vi "Lab Panel V5.25.vi"() -> ()   [LabVIEW 2017] (continued)
                        n582 = Unbundle(w867) -> ("AMPS"=w870:dbl)  [unwired: 4 out]
                        n583 = call "Check For Amps on v1.vi"("ID"="LAB01-2", "amps"=w870) -> ("amps"=w868:bool)  [unwired: 9 in]
                      }
                      frame #1 {
                        n584 = case shown="True" w872 {
                          tunnel: w882 -> [_ w895]
                          tunnel: w881 -> [_ w894]
                          tunnel: w880 -> [_ w893]
                          tunnel: w879 -> [_ w892]
                          tunnel: w878 -> [_ w891]
                          tunnel: [errorcluster {"status"=FALSE, "code"=0, "source"=""} ("error out") w890] -> w877
                          tunnel: w876 -> [_ w889]
                          tunnel: w875 -> [_ w888]
                          tunnel: w874 -> [_ w887]
                          tunnel: w873 -> [_ w886]
                          tunnel: w871 -> [_ w885]
                          frame False {
                            w883 = FALSE
                            n585 = local write "RUN LAB01-2"(w883) -> ()
                            n586 = local write "run lab01-2"(w883) -> ()
                          }
                          frame True {
                            n587 = stacked-sequence {
                              seq-local: [w896 _ _ _ _] -> [_ w920 _ _ _]
                              tunnel: w895 -> [w901 _ _ _ _]
                              tunnel: w894 -> [w898 _ _ _ _]
                              tunnel: w893 -> [w911 _ _ _ _]
                              tunnel: w892 -> [w904 _ _ _ _]
                              tunnel: w891 -> [w899 _ _ _ _]
                              tunnel: [_ w915 _ _ _] -> w890
                              tunnel: w889 -> [_ _ _ w942 _]
                              tunnel: w888 -> [_ _ _ w941 _]
                              tunnel: w887 -> [_ _ _ w940 _]
                              tunnel: w886 -> [_ _ _ _ _]
                              tunnel: w885 -> [_ _ _ _ w955]
                              frame #0 {
                                w897 = "\\"
                                n588 = local read "SET LAB01-2"() -> (w906:T5)
                                n589 = case shown="\"CYCLE TEST\"" w911 {
                                tunnel: ["L01-2-CHART TEST-" "L01-2-CYCLE TEST-" "L01-2-T-RISE TEST-"] -> w907
                                frame "CHART TEST", Default {
                                }
                                frame "CYCLE TEST" {
                                }
                                frame "T-RISE TEST" {
                                }
                                }
                                n590 = Unbundle(w906) -> ("DESCRIPTION"=w905:string)  [unwired: 4 out]
                                n591 = Concatenate Strings(w901, "\\", w899, w897, w898, w897) -> (w908:string)
                                n592 = String To Path(string=w908) -> (path=w910:path)
                                n593 = Concatenate Strings(w908, w907, w905, "-", w904, ".tdms") -> (w896:string)
                                n594 = Create Folder(path (use dialog)=w910) -> (error out=w909:errorcluster)  [unwired: 2 in, 2 out]
                                n595 = call <vilib>:"Clear Errors.vi"("error in (no error)"=w909) -> ()  [unwired: 5 in, 2 out]
                                n596 = global write "Global 1.vi" "LAB01-2 FILE"(w896) -> ()
                              }
                              frame #1 {
                                (unwired) FALSE
                                n597 = String To Path(string=w920) -> (path=w916:path)
                                n598 = TDMS Open(6:FALSE, 10:T21."create or replace" ("operation (0:open)"), 11:w916) -> (0:w915:errorcluster, 3:→"TDMS LAB01-2":refnum<k34>)  [unwired: 4 in]
                              }
                              frame #2 {
                                n599 = local read "SET LAB01-2"() -> (w926:T5)
                                n600 = local read "TDMS LAB01-2"() -> (w937:refnum<k34>)
                                n601 = Build Array("Testers Name", "Description", "Set Test Cycles", "T-Rise minutes", "T-Rise Deg C") -> (w927:string[])
                                n602 = Unbundle(w926) -> ("NAME"=w925:string, "DESCRIPTION"=w924:string, "CYCLES"=w923:dbl, "T-RISE mins"=w922:dbl, "T-RISE deg C"=w921:dbl)
                                n603 = Number To Decimal String(number=w923) -> (decimal integer string=w936:string)  [unwired: 1 in]
                                n604 = Number To Decimal String(number=w922) -> (decimal integer string=w935:string)  [unwired: 1 in]
                                n605 = Number To Decimal String(number=w921) -> (decimal integer string=w934:string)  [unwired: 1 in]
                                n606 = Build Array(w925, w924, w936, w935, w934) -> (w933:string[])
                                n607 = TDMS Set Properties(5:w933, 7:w927, 11:w937) -> ()  [unwired: 3 in, 4 out]
                              }
                              frame #3 {
                                n608 = local read "DISP LAB01-2"() -> (w939:T4)
                                n609 = Concatenate Strings("LAB01-2  ", w942) -> (w943:string)
                                n610 = Two Button Dialog(message=w943, 1:w940, 2:w941) -> (T button?=w945:bool)
                                n611 = case shown="True" w945 {
                                tunnel: w939 -> [w952 w953]
                                tunnel: [w952 w953] -> w949
                                tunnel: [w951 w954] -> w948
                                tunnel: [w950 w954] -> w947
                                frame False {
                                n612 = Unbundle(w952) -> ("CYCLE"=w951:dbl, "MINS"=w950:dbl)  [unwired: 1 out]
                                }
                                frame True {
                                w954 = 0.0
                                }
                                }
                                n613 = Bundle(cluster=w949, "CYCLE"=w948, "MINS"=w947, "STATUS"="RUN") -> (w938:T4)
                                n614 = local write "DISP LAB01-2"(w938) -> ()
                              }
                              frame #4 {
                                n615 = local read "TEMP START LAB01-2"() -> (w957:cluster{"TL":dbl, "TN":dbl})
                                n616 = Bundle(cluster=w957, "TL"=w955, "TN"=w955) -> (w956:cluster{"TL":dbl, "TN":dbl})
                                n617 = local write "TEMP START LAB01-2"(w956) -> ()
                              }
                            }
                          }
                        }
                      }
                    }
                  }
                }
              }
              event "RUN LAB02-1": Value Change {
                n618 = event-data() -> ("NewVal"=w963:bool)  [unwired: 1 in, 5 out]
                n619 = local read "SIG LAB02-1"() -> (w959:T2)
                n620 = case shown="True" w963 {
                  tunnel: w969 -> [_ w1007]
                  tunnel: w968 -> [_ w1006]
                  tunnel: w966 -> [w971 w1005]
                  tunnel: w967 -> [_ w1004]
                  tunnel: w965 -> [_ w1003]
                  tunnel: [w970 w1002] -> w964
                  tunnel: w962 -> [_ w1001]
                  tunnel: w961 -> [_ w1000]
                  tunnel: w960 -> [_ w999]
                  tunnel: w959 -> [_ w998]
                  tunnel: w958 -> [_ w997]
                  frame False {
                    # "stop test"
                    n621 = stacked-sequence {
                      tunnel: w971 -> [w980 _]
                      tunnel: [w972 _] -> w970
                      frame #0 {
                        n622 = local read "DISP LAB02-1"() -> (w979:T4)
                        n623 = Unbundle(w979) -> ("CYCLE"=w977:dbl, "MINS"=w978:dbl)  [unwired: 1 out]
                        n624 = case shown="\"CYCLE TEST\"" w980 {
                          tunnel: w978 -> [_ _ w987]
                          tunnel: w977 -> [w985 w986 _]
                          tunnel: [w985 w986 w987] -> w976
                          frame "CHART TEST", Default {
                          }
                          frame "CYCLE TEST" {
                          }
                          frame "T-RISE TEST" {
                          }
                        }
                        n625 = local read "TDMS LAB02-1"() -> (w984:refnum<k34>)
                        n626 = Build Array("STOPPED") -> (w981:string[])
                        n627 = Build Array(w976) -> (w975:dbl[])
                        n628 = TDMS Write(0:w984, 5:"TEST RESULT", 7:w981, 9:w975) -> (4:w973:refnum<k34>, 15:w974:errorcluster)  [unwired: 2 in, 2 out]
                        n629 = TDMS Close(8:w974, 11:w973) -> (0:w972:errorcluster)  [unwired: 1 out]
                      }
                      frame #1 {
                        n630 = local read "DISP LAB02-1"() -> (w991:T4)
                        n631 = stacked-sequence {
                          tunnel: "LAB02-1" -> [w993 w995]
                          frame #0 {
                            n632 = call "sub vi - defrag tdms v1.vi"("panel id"=w993) -> ("error out"=w992:errorcluster)  [unwired: 10 in]
                            n633 = local write "data file error"(w992) -> ()
                          }
                          frame #1 {
                            n634 = local write "RESULT LAB02-1"(FALSE) -> ()
                            n635 = call "Save data file (stop) v3.vi"("panel id"=w995) -> ("network file save error"=w994:errorcluster)  [unwired: 9 in, 1 out]
                            n636 = local write "data file error"(w994) -> ()
                          }
                        }
                        n637 = Bundle(cluster=w991, "STATUS"="STOP") -> (w989:T4)  [unwired: 2 in]
                        n638 = local write "DISP LAB02-1"(w989) -> ()
                      }
                    }
                  }
                  frame True {
                    n639 = stacked-sequence {
                      seq-local: [w1009 _] -> [_ w1013]
                      tunnel: w1007 -> [_ w1023]
                      tunnel: w1006 -> [_ w1022]
                      tunnel: w1005 -> [_ w1021]
                      tunnel: w1004 -> [_ w1020]
                      tunnel: w1003 -> [_ w1019]
                      tunnel: [_ w1018] -> w1002
                      tunnel: w1001 -> [_ w1017]
                      tunnel: w1000 -> [_ w1016]
                      tunnel: w999 -> [_ w1015]
                      tunnel: w998 -> [w1008 w1014]
                      tunnel: w997 -> [_ w1012]
                      frame #0 {
                        n640 = Unbundle(w1008) -> ("AMPS"=w1011:dbl)  [unwired: 4 out]
                        n641 = call "Check For Amps on v1.vi"("ID"="LAB02-1", "amps"=w1011) -> ("amps"=w1009:bool)  [unwired: 9 in]
                      }
                      frame #1 {
                        n642 = case shown="True" w1013 {
                          tunnel: w1023 -> [_ w1036]
                          tunnel: w1022 -> [_ w1035]
                          tunnel: w1021 -> [_ w1034]
                          tunnel: w1020 -> [_ w1033]
                          tunnel: w1019 -> [_ w1032]
                          tunnel: [errorcluster {"status"=FALSE, "code"=0, "source"=""} ("error out") w1031] -> w1018
                          tunnel: w1017 -> [_ w1030]
                          tunnel: w1016 -> [_ w1029]
                          tunnel: w1015 -> [_ w1028]
                          tunnel: w1014 -> [_ w1027]
                          tunnel: w1012 -> [_ w1026]
                          frame False {
                            w1025 = FALSE
                            n643 = local write "RUN LAB02-1"(w1025) -> ()
                            n644 = local write "run lab02-1"(w1025) -> ()
                          }
                          frame True {
                            n645 = stacked-sequence {
                              seq-local: [w1037 _ _ _ _] -> [_ w1061 _ _ _]
                              tunnel: w1036 -> [w1042 _ _ _ _]
                              tunnel: w1035 -> [w1039 _ _ _ _]
                              tunnel: w1034 -> [w1052 _ _ _ _]
                              tunnel: w1033 -> [w1045 _ _ _ _]
                              tunnel: w1032 -> [w1040 _ _ _ _]
                              tunnel: [_ w1056 _ _ _] -> w1031
                              tunnel: w1030 -> [_ _ _ w1082 _]
                              tunnel: w1029 -> [_ _ _ w1081 _]
                              tunnel: w1028 -> [_ _ _ w1080 _]
                              tunnel: w1027 -> [_ _ _ _ _]
                              tunnel: w1026 -> [_ _ _ _ w1096]
                              frame #0 {
                                w1038 = "\\"
                                n646 = local read "SET LAB02-1"() -> (w1047:T5)
                                n647 = case shown="\"CYCLE TEST\"" w1052 {
                                tunnel: ["L02-1-CHART TEST-" "L02-1-CYCLE TEST-" "L02-1-T-RISE TEST-"] -> w1048
                                frame "CHART TEST", Default {
                                }
                                frame "CYCLE TEST" {
                                }
                                frame "T-RISE TEST" {
                                }
                                }
                                n648 = Unbundle(w1047) -> ("DESCRIPTION"=w1046:string)  [unwired: 4 out]
                                n649 = Concatenate Strings(w1042, "\\", w1040, w1038, w1039, w1038) -> (w1049:string)
                                n650 = String To Path(string=w1049) -> (path=w1051:path)
                                n651 = Concatenate Strings(w1049, w1048, w1046, "-", w1045, ".tdms") -> (w1037:string)
                                n652 = Create Folder(path (use dialog)=w1051) -> (error out=w1050:errorcluster)  [unwired: 2 in, 2 out]
                                n653 = global write "Global 1.vi" "LAB02-1 FILE"(w1037) -> ()
                                n654 = call <vilib>:"Clear Errors.vi"("error in (no error)"=w1050) -> ()  [unwired: 5 in, 2 out]
                              }
                              frame #1 {
                                (unwired) FALSE
                                n655 = String To Path(string=w1061) -> (path=w1057:path)
                                n656 = TDMS Open(6:FALSE, 10:T21."create or replace" ("operation (0:open)"), 11:w1057) -> (0:w1056:errorcluster, 3:→"TDMS LAB02-1":refnum<k34>)  [unwired: 4 in]
                              }
                              frame #2 {
                                n657 = local read "SET LAB02-1"() -> (w1067:T5)
                                n658 = local read "TDMS LAB02-1"() -> (w1078:refnum<k34>)
                                n659 = Build Array("Testers Name", "Description", "Set Test Cycles", "T-Rise minutes", "T-Rise Deg C") -> (w1068:string[])
                                n660 = Unbundle(w1067) -> ("NAME"=w1066:string, "DESCRIPTION"=w1065:string, "CYCLES"=w1064:dbl, "T-RISE mins"=w1063:dbl, "T-RISE deg C"=w1062:dbl)
                                n661 = Number To Decimal String(number=w1064) -> (decimal integer string=w1077:string)  [unwired: 1 in]
                                n662 = Number To Decimal String(number=w1063) -> (decimal integer string=w1076:string)  [unwired: 1 in]
                                n663 = Number To Decimal String(number=w1062) -> (decimal integer string=w1075:string)  [unwired: 1 in]
                                n664 = Build Array(w1066, w1065, w1077, w1076, w1075) -> (w1074:string[])
                                n665 = TDMS Set Properties(5:w1074, 7:w1068, 11:w1078) -> ()  [unwired: 3 in, 4 out]
                              }
                              frame #3 {
                                n666 = local read "DISP LAB02-1"() -> (w1083:T4)
                                n667 = Concatenate Strings("LAB02-1  ", w1082) -> (w1084:string)
                                n668 = Two Button Dialog(message=w1084, 1:w1080, 2:w1081) -> (T button?=w1086:bool)
                                n669 = case shown="True" w1086 {
                                tunnel: w1083 -> [w1093 w1094]
                                tunnel: [w1093 w1094] -> w1090
                                tunnel: [w1092 w1095] -> w1089
                                tunnel: [w1091 w1095] -> w1088
                                frame False {
                                n670 = Unbundle(w1093) -> ("CYCLE"=w1092:dbl, "MINS"=w1091:dbl)  [unwired: 1 out]
                                }
                                frame True {
                                w1095 = 0.0
                                }
                                }
                                n671 = Bundle(cluster=w1090, "CYCLE"=w1089, "MINS"=w1088, "STATUS"="RUN") -> (w1079:T4)
                                n672 = local write "DISP LAB02-1"(w1079) -> ()
                              }
                              frame #4 {
                                n673 = local read "TEMP START LAB02-1"() -> (w1098:cluster{"TL":dbl, "TN":dbl})
                                n674 = Bundle(cluster=w1098, "TL"=w1096, "TN"=w1096) -> (w1097:cluster{"TL":dbl, "TN":dbl})
                                n675 = local write "TEMP START LAB02-1"(w1097) -> ()
                              }
                            }
                          }
                        }
                      }
                    }
                  }
                }
                n676 = local write "run lab02-1"(w963) -> ()
              }
              event "RUN LAB02-2": Value Change {
                n677 = event-data() -> ("NewVal"=w1103:bool)  [unwired: 1 in, 5 out]
                n678 = local write "run lab02-2"(w1103) -> ()
                n679 = case shown="True" w1103 {
                  tunnel: w1109 -> [_ w1147]
                  tunnel: w1108 -> [_ w1146]
                  tunnel: w1106 -> [w1111 w1145]
                  tunnel: w1107 -> [_ w1144]
                  tunnel: w1105 -> [_ w1143]
                  tunnel: [w1110 w1142] -> w1104
                  tunnel: w1102 -> [_ w1141]
                  tunnel: w1101 -> [_ w1140]
                  tunnel: w1100 -> [_ w1139]
                  tunnel: w1099 -> [_ w1137]
                  frame False {
                    # "stop test"
                    n680 = stacked-sequence {
                      tunnel: w1111 -> [w1120 _]
                      tunnel: [w1112 _] -> w1110
                      frame #0 {
                        n681 = local read "DISP LAB02-2"() -> (w1119:T4)
                        n682 = Unbundle(w1119) -> ("CYCLE"=w1117:dbl, "MINS"=w1118:dbl)  [unwired: 1 out]
                        n683 = case shown="\"CYCLE TEST\"" w1120 {
                          tunnel: w1118 -> [_ _ w1127]
                          tunnel: w1117 -> [w1125 w1126 _]
                          tunnel: [w1125 w1126 w1127] -> w1116
                          frame "CHART TEST", Default {
                          }
                          frame "CYCLE TEST" {
                          }
                          frame "T-RISE TEST" {
                          }
                        }
                        n684 = local read "TDMS LAB02-2"() -> (w1124:refnum<k34>)
                        n685 = Build Array("STOPPED") -> (w1121:string[])
                        n686 = Build Array(w1116) -> (w1115:dbl[])
                        n687 = TDMS Write(0:w1124, 5:"TEST RESULT", 7:w1121, 9:w1115) -> (4:w1113:refnum<k34>, 15:w1114:errorcluster)  [unwired: 2 in, 2 out]
                        n688 = TDMS Close(8:w1114, 11:w1113) -> (0:w1112:errorcluster)  [unwired: 1 out]
                      }
                      frame #1 {
                        n689 = local read "DISP LAB02-2"() -> (w1131:T4)
                        n690 = stacked-sequence {
                          tunnel: "LAB02-2" -> [w1133 w1135]
                          frame #0 {
                            n691 = call "sub vi - defrag tdms v1.vi"("panel id"=w1133) -> ("error out"=w1132:errorcluster)  [unwired: 10 in]
                            n692 = local write "data file error"(w1132) -> ()
                          }
                          frame #1 {
                            n693 = call "Save data file (stop) v3.vi"("panel id"=w1135) -> ("network file save error"=w1134:errorcluster)  [unwired: 9 in, 1 out]
                            n694 = local write "RESULT LAB02-2"(FALSE) -> ()
                            n695 = local write "data file error"(w1134) -> ()
                          }
                        }
                        n696 = Bundle(cluster=w1131, "STATUS"="STOP") -> (w1129:T4)  [unwired: 2 in]
                        n697 = local write "DISP LAB02-2"(w1129) -> ()
                      }
                    }
                  }
                  frame True {
                    n698 = local read "SIG LAB02-2"() -> (w1138:T2)
                    n699 = stacked-sequence {
                      seq-local: [w1149 _] -> [_ w1153]
                      tunnel: w1147 -> [_ w1163]
                      tunnel: w1146 -> [_ w1162]
                      tunnel: w1145 -> [_ w1161]
                      tunnel: w1144 -> [_ w1160]
                      tunnel: w1143 -> [_ w1159]
                      tunnel: [_ w1158] -> w1142
                      tunnel: w1141 -> [_ w1157]
                      tunnel: w1140 -> [_ w1156]
                      tunnel: w1139 -> [_ w1155]
                      tunnel: w1138 -> [w1148 w1154]
                      tunnel: w1137 -> [_ w1152]
                      frame #0 {
                        n700 = Unbundle(w1148) -> ("AMPS"=w1151:dbl)  [unwired: 4 out]
                        n701 = call "Check For Amps on v1.vi"("ID"="LAB02-2", "amps"=w1151) -> ("amps"=w1149:bool)  [unwired: 9 in]
                      }
                      frame #1 {
                        n702 = case shown="True" w1153 {
                          tunnel: w1163 -> [_ w1176]
                          tunnel: w1162 -> [_ w1175]
                          tunnel: w1161 -> [_ w1174]
                          tunnel: w1160 -> [_ w1173]
                          tunnel: w1159 -> [_ w1172]
                          tunnel: [errorcluster {"status"=FALSE, "code"=0, "source"=""} ("error out") w1171] -> w1158
                          tunnel: w1157 -> [_ w1170]
                          tunnel: w1156 -> [_ w1169]
                          tunnel: w1155 -> [_ w1168]
                          tunnel: w1154 -> [_ w1167]
                          tunnel: w1152 -> [_ w1166]
                          frame False {
                            w1164 = FALSE
                            n703 = local write "RUN LAB02-2"(w1164) -> ()
                            n704 = local write "run lab02-2"(w1164) -> ()
                          }
                          frame True {
                            n705 = stacked-sequence {
                              seq-local: [w1177 _ _ _ _] -> [_ w1201 _ _ _]
                              tunnel: w1176 -> [w1182 _ _ _ _]
                              tunnel: w1175 -> [w1179 _ _ _ _]
                              tunnel: w1174 -> [w1192 _ _ _ _]
                              tunnel: w1173 -> [w1185 _ _ _ _]
                              tunnel: w1172 -> [w1180 _ _ _ _]
                              tunnel: [_ w1196 _ _ _] -> w1171
                              tunnel: w1170 -> [_ _ _ w1222 _]
                              tunnel: w1169 -> [_ _ _ w1221 _]
                              tunnel: w1168 -> [_ _ _ w1220 _]
                              tunnel: w1167 -> [_ _ _ _ _]
                              tunnel: w1166 -> [_ _ _ _ w1236]
                              frame #0 {
                                w1178 = "\\"
                                n706 = local read "SET LAB02-2"() -> (w1187:T5)
                                n707 = case shown="\"CYCLE TEST\"" w1192 {
                                tunnel: ["L02-2-CHART TEST-" "L02-2-CYCLE TEST-" "L02-2-T-RISE TEST-"] -> w1188
                                frame "CHART TEST", Default {
                                }
                                frame "CYCLE TEST" {
                                }
                                frame "T-RISE TEST" {
                                }
                                }
                                n708 = Unbundle(w1187) -> ("DESCRIPTION"=w1186:string)  [unwired: 4 out]
                                n709 = Concatenate Strings(w1182, "\\", w1180, w1178, w1179, w1178) -> (w1189:string)
                                n710 = String To Path(string=w1189) -> (path=w1191:path)
                                n711 = Concatenate Strings(w1189, w1188, w1186, "-", w1185, ".tdms") -> (w1177:string)
                                n712 = Create Folder(path (use dialog)=w1191) -> (error out=w1190:errorcluster)  [unwired: 2 in, 2 out]
                                n713 = global write "Global 1.vi" "LAB02-2 FILE"(w1177) -> ()
                                n714 = call <vilib>:"Clear Errors.vi"("error in (no error)"=w1190) -> ()  [unwired: 5 in, 2 out]
                              }
                              frame #1 {
                                (unwired) FALSE
                                n715 = String To Path(string=w1201) -> (path=w1197:path)
                                n716 = TDMS Open(6:FALSE, 10:T21."create or replace" ("operation (0:open)"), 11:w1197) -> (0:w1196:errorcluster, 3:→"TDMS LAB02-2":refnum<k34>)  [unwired: 4 in]
                              }
                              frame #2 {
                                n717 = local read "SET LAB02-2"() -> (w1207:T5)
                                n718 = local read "TDMS LAB02-2"() -> (w1218:refnum<k34>)
                                n719 = Build Array("Testers Name", "Description", "Set Test Cycles", "T-Rise minutes", "T-Rise Deg C") -> (w1208:string[])
                                n720 = Unbundle(w1207) -> ("NAME"=w1206:string, "DESCRIPTION"=w1205:string, "CYCLES"=w1204:dbl, "T-RISE mins"=w1203:dbl, "T-RISE deg C"=w1202:dbl)
                                n721 = Number To Decimal String(number=w1204) -> (decimal integer string=w1217:string)  [unwired: 1 in]
                                n722 = Number To Decimal String(number=w1203) -> (decimal integer string=w1216:string)  [unwired: 1 in]
                                n723 = Number To Decimal String(number=w1202) -> (decimal integer string=w1215:string)  [unwired: 1 in]
                                n724 = Build Array(w1206, w1205, w1217, w1216, w1215) -> (w1214:string[])
                                n725 = TDMS Set Properties(5:w1214, 7:w1208, 11:w1218) -> ()  [unwired: 3 in, 4 out]
                              }
                              frame #3 {
                                n726 = local read "DISP LAB02-2"() -> (w1223:T4)
                                n727 = Concatenate Strings("LAB02-2  ", w1222) -> (w1224:string)
                                n728 = Two Button Dialog(message=w1224, 1:w1220, 2:w1221) -> (T button?=w1226:bool)
                                n729 = case shown="True" w1226 {
                                tunnel: w1223 -> [w1233 w1234]
                                tunnel: [w1233 w1234] -> w1230
                                tunnel: [w1232 w1235] -> w1229
                                tunnel: [w1231 w1235] -> w1228
                                frame False {
                                n730 = Unbundle(w1233) -> ("CYCLE"=w1232:dbl, "MINS"=w1231:dbl)  [unwired: 1 out]
                                }
                                frame True {
                                w1235 = 0.0
                                }
                                }
                                n731 = Bundle(cluster=w1230, "CYCLE"=w1229, "MINS"=w1228, "STATUS"="RUN") -> (w1219:T4)
                                n732 = local write "DISP LAB02-2"(w1219) -> ()
                              }
                              frame #4 {
                                n733 = local read "TEMP START LAB02-2"() -> (w1238:cluster{"TL":dbl, "TN":dbl})
                                n734 = Bundle(cluster=w1238, "TL"=w1236, "TN"=w1236) -> (w1237:cluster{"TL":dbl, "TN":dbl})
                                n735 = local write "TEMP START LAB02-2"(w1237) -> ()
                              }
                            }
                          }
                        }
                      }
                    }
                  }
                }
              }
              event "RUN LAB03-1": Value Change {
                n736 = event-data() -> ("NewVal"=w1243:bool)  [unwired: 1 in, 5 out]
                n737 = local write "run lab03-1"(w1243) -> ()
                n738 = case shown="True" w1243 {
                  tunnel: w1249 -> [_ w1287]
                  tunnel: w1248 -> [_ w1286]
                  tunnel: w1246 -> [w1251 w1285]
                  tunnel: w1247 -> [_ w1284]
                  tunnel: w1245 -> [_ w1283]
                  tunnel: [w1250 w1282] -> w1244
                  tunnel: w1242 -> [_ w1281]
                  tunnel: w1241 -> [_ w1280]
                  tunnel: w1240 -> [_ w1279]
                  tunnel: w1239 -> [_ w1277]
                  frame False {
                    # "stop test"
                    n739 = stacked-sequence {
                      tunnel: w1251 -> [w1260 _]
                      tunnel: [w1252 _] -> w1250
                      frame #0 {
                        n740 = local read "DISP LAB03-1"() -> (w1259:T4)
                        n741 = Unbundle(w1259) -> ("CYCLE"=w1257:dbl, "MINS"=w1258:dbl)  [unwired: 1 out]
                        n742 = case shown="\"CYCLE TEST\"" w1260 {
                          tunnel: w1258 -> [_ _ w1267]
                          tunnel: w1257 -> [w1265 w1266 _]
                          tunnel: [w1265 w1266 w1267] -> w1256
                          frame "CHART TEST", Default {
                          }
                          frame "CYCLE TEST" {
                          }
                          frame "T-RISE TEST" {
                          }
                        }
                        n743 = local read "TDMS LAB03-1"() -> (w1264:refnum<k34>)
                        n744 = Build Array("STOPPED") -> (w1261:string[])
                        n745 = Build Array(w1256) -> (w1255:dbl[])
                        n746 = TDMS Write(0:w1264, 5:"TEST RESULT", 7:w1261, 9:w1255) -> (4:w1253:refnum<k34>, 15:w1254:errorcluster)  [unwired: 2 in, 2 out]
                        n747 = TDMS Close(8:w1254, 11:w1253) -> (0:w1252:errorcluster)  [unwired: 1 out]
                      }
                      frame #1 {
                        n748 = local read "DISP LAB03-1"() -> (w1271:T4)
                        n749 = stacked-sequence {
                          tunnel: "LAB03-1" -> [w1273 w1275]
                          frame #0 {
                            n750 = call "sub vi - defrag tdms v1.vi"("panel id"=w1273) -> ("error out"=w1272:errorcluster)  [unwired: 10 in]
                            n751 = local write "data file error"(w1272) -> ()
                          }
                          frame #1 {
                            n752 = call "Save data file (stop) v3.vi"("panel id"=w1275) -> ("network file save error"=w1274:errorcluster)  [unwired: 9 in, 1 out]
                            n753 = local write "RESULT LAB03-1"(FALSE) -> ()
                            n754 = local write "data file error"(w1274) -> ()
                          }
                        }
                        n755 = Bundle(cluster=w1271, "STATUS"="STOP") -> (w1269:T4)  [unwired: 2 in]
                        n756 = local write "DISP LAB03-1"(w1269) -> ()
                      }
                    }
                  }
                  frame True {
                    n757 = local read "SIG LAB03-1"() -> (w1278:T2)
                    n758 = stacked-sequence {
                      seq-local: [w1289 _] -> [_ w1293]
                      tunnel: w1287 -> [_ w1303]
                      tunnel: w1286 -> [_ w1302]
                      tunnel: w1285 -> [_ w1301]
                      tunnel: w1284 -> [_ w1300]
                      tunnel: w1283 -> [_ w1299]
                      tunnel: [_ w1298] -> w1282
                      tunnel: w1281 -> [_ w1297]
                      tunnel: w1280 -> [_ w1296]
                      tunnel: w1279 -> [_ w1295]
                      tunnel: w1278 -> [w1288 w1294]
                      tunnel: w1277 -> [_ w1292]
                      frame #0 {
                        n759 = Unbundle(w1288) -> ("AMPS"=w1291:dbl)  [unwired: 4 out]
                        n760 = call "Check For Amps on v1.vi"("ID"="LAB03-1", "amps"=w1291) -> ("amps"=w1289:bool)  [unwired: 9 in]
                      }
                      frame #1 {
                        n761 = case shown="True" w1293 {
                          tunnel: w1303 -> [_ w1316]
                          tunnel: w1302 -> [_ w1315]
                          tunnel: w1301 -> [_ w1314]
                          tunnel: w1300 -> [_ w1313]
                          tunnel: w1299 -> [_ w1312]
                          tunnel: [errorcluster {"status"=FALSE, "code"=0, "source"=""} ("error out") w1311] -> w1298
                          tunnel: w1297 -> [_ w1310]
                          tunnel: w1296 -> [_ w1309]
                          tunnel: w1295 -> [_ w1308]
                          tunnel: w1294 -> [_ w1307]
                          tunnel: w1292 -> [_ w1306]
                          frame False {
                            w1304 = FALSE
                            n762 = local write "RUN LAB03-1"(w1304) -> ()
                            n763 = local write "run lab03-1"(w1304) -> ()
                          }
                          frame True {
                            n764 = stacked-sequence {
                              seq-local: [w1317 _ _ _ _] -> [_ w1341 _ _ _]
                              tunnel: w1316 -> [w1322 _ _ _ _]
                              tunnel: w1315 -> [w1319 _ _ _ _]
                              tunnel: w1314 -> [w1332 _ _ _ _]
                              tunnel: w1313 -> [w1325 _ _ _ _]
                              tunnel: w1312 -> [w1320 _ _ _ _]
                              tunnel: [_ w1336 _ _ _] -> w1311
                              tunnel: w1310 -> [_ _ _ w1361 _]
                              tunnel: w1309 -> [_ _ _ w1360 _]
                              tunnel: w1308 -> [_ _ _ w1359 _]
                              tunnel: w1307 -> [_ _ _ _ _]
                              tunnel: w1306 -> [_ _ _ _ w1376]
                              frame #0 {
                                w1318 = "\\"
                                n765 = local read "SET LAB03-1"() -> (w1327:T5)
                                n766 = case shown="\"T-RISE TEST\"" w1332 {
                                tunnel: ["L03-1-CHART TEST-" "L03-1-CYCLE TEST-" "L03-1-T-RISE TEST-"] -> w1328
                                frame "CHART TEST", Default {
                                }
                                frame "CYCLE TEST" {
                                }
                                frame "T-RISE TEST" {
                                }
                                }
                                n767 = Unbundle(w1327) -> ("DESCRIPTION"=w1326:string)  [unwired: 4 out]
                                n768 = Concatenate Strings(w1322, "\\", w1320, w1318, w1319, w1318) -> (w1329:string)
                                n769 = String To Path(string=w1329) -> (path=w1331:path)
                                n770 = Concatenate Strings(w1329, w1328, w1326, "-", w1325, ".tdms") -> (w1317:string)
                                n771 = Create Folder(path (use dialog)=w1331) -> (error out=w1330:errorcluster)  [unwired: 2 in, 2 out]
                                n772 = global write "Global 1.vi" "LAB03-1 FILE"(w1317) -> ()
                                n773 = call <vilib>:"Clear Errors.vi"("error in (no error)"=w1330) -> ()  [unwired: 5 in, 2 out]
                              }
                              frame #1 {
                                (unwired) FALSE
                                n774 = String To Path(string=w1341) -> (path=w1337:path)
                                n775 = TDMS Open(6:FALSE, 10:T21."create or replace" ("operation (0:open)"), 11:w1337) -> (0:w1336:errorcluster, 3:→"TDMS LAB03-1":refnum<k34>)  [unwired: 4 in]
                              }
                              frame #2 {
                                n776 = local read "SET LAB03-1"() -> (w1347:T5)
                                n777 = local read "TDMS LAB03-1"() -> (w1358:refnum<k34>)
                                n778 = Build Array("Testers Name", "Description", "Set Test Cycles", "T-Rise minutes", "T-Rise Deg C") -> (w1348:string[])
                                n779 = Unbundle(w1347) -> ("NAME"=w1346:string, "DESCRIPTION"=w1345:string, "CYCLES"=w1344:dbl, "T-RISE mins"=w1343:dbl, "T-RISE deg C"=w1342:dbl)
                                n780 = Number To Decimal String(number=w1344) -> (decimal integer string=w1357:string)  [unwired: 1 in]
                                n781 = Number To Decimal String(number=w1343) -> (decimal integer string=w1356:string)  [unwired: 1 in]
                                n782 = Number To Decimal String(number=w1342) -> (decimal integer string=w1355:string)  [unwired: 1 in]
                                n783 = Build Array(w1346, w1345, w1357, w1356, w1355) -> (w1354:string[])
                                n784 = TDMS Set Properties(5:w1354, 7:w1348, 11:w1358) -> ()  [unwired: 3 in, 4 out]
                              }
                              frame #3 {
                                n785 = local read "DISP LAB03-1"() -> (w1363:T4)
                                n786 = Concatenate Strings("LAB03-1  ", w1361) -> (w1364:string)
                                n787 = Two Button Dialog(message=w1364, 1:w1359, 2:w1360) -> (T button?=w1366:bool)
                                n788 = case shown="True" w1366 {
                                tunnel: w1363 -> [w1373 w1374]
                                tunnel: [w1373 w1374] -> w1370
                                tunnel: [w1372 w1375] -> w1369
                                tunnel: [w1371 w1375] -> w1368
                                frame False {
                                n789 = Unbundle(w1373) -> ("CYCLE"=w1372:dbl, "MINS"=w1371:dbl)  [unwired: 1 out]
                                }
                                frame True {
                                w1375 = 0.0
                                }
                                }
                                n790 = Bundle(cluster=w1370, "CYCLE"=w1369, "MINS"=w1368, "STATUS"="RUN") -> (w1362:T4)
                                n791 = local write "DISP LAB03-1"(w1362) -> ()
                              }
                              frame #4 {
                                n792 = local read "TEMP START LAB03-1"() -> (w1378:cluster{"TL":dbl, "TN":dbl})
                                n793 = Bundle(cluster=w1378, "TL"=w1376, "TN"=w1376) -> (w1377:cluster{"TL":dbl, "TN":dbl})
                                n794 = local write "TEMP START LAB03-1"(w1377) -> ()
                              }
                            }
                          }
                        }
                      }
                    }
                  }
                }
              }
              event "RUN LAB03-2": Value Change {
                n795 = event-data() -> ("NewVal"=w1383:bool)  [unwired: 1 in, 5 out]
                n796 = local write "run lab03-2"(w1383) -> ()
                n797 = case shown="True" w1383 {
                  tunnel: w1389 -> [_ w1427]
                  tunnel: w1388 -> [_ w1426]
                  tunnel: w1386 -> [w1391 w1425]
                  tunnel: w1387 -> [_ w1424]
                  tunnel: w1385 -> [_ w1423]
                  tunnel: [w1390 w1422] -> w1384
                  tunnel: w1382 -> [_ w1421]
                  tunnel: w1381 -> [_ w1420]
                  tunnel: w1380 -> [_ w1419]
                  tunnel: w1379 -> [_ w1417]
                  frame False {
                    # "stop test"
                    n798 = stacked-sequence {
                      tunnel: w1391 -> [w1400 _]
                      tunnel: [w1392 _] -> w1390
                      frame #0 {
                        n799 = local read "DISP LAB03-2"() -> (w1399:T4)
                        n800 = Unbundle(w1399) -> ("CYCLE"=w1397:dbl, "MINS"=w1398:dbl)  [unwired: 1 out]
                        n801 = case shown="\"CYCLE TEST\"" w1400 {
                          tunnel: w1398 -> [_ _ w1407]
                          tunnel: w1397 -> [w1405 w1406 _]
                          tunnel: [w1405 w1406 w1407] -> w1396
                          frame "CHART TEST", Default {
                          }
                          frame "CYCLE TEST" {
                          }
                          frame "T-RISE TEST" {
                          }
                        }
                        n802 = local read "TDMS LAB03-2"() -> (w1404:refnum<k34>)
                        n803 = Build Array("STOPPED") -> (w1401:string[])
                        n804 = Build Array(w1396) -> (w1395:dbl[])
                        n805 = TDMS Write(0:w1404, 5:"TEST RESULT", 7:w1401, 9:w1395) -> (4:w1393:refnum<k34>, 15:w1394:errorcluster)  [unwired: 2 in, 2 out]
                        n806 = TDMS Close(8:w1394, 11:w1393) -> (0:w1392:errorcluster)  [unwired: 1 out]
                      }
                      frame #1 {
                        n807 = local read "DISP LAB03-2"() -> (w1411:T4)
                        n808 = stacked-sequence {
                          tunnel: "LAB03-2" -> [w1413 w1415]
                          frame #0 {
                            n809 = call "sub vi - defrag tdms v1.vi"("panel id"=w1413) -> ("error out"=w1412:errorcluster)  [unwired: 10 in]
                            n810 = local write "data file error"(w1412) -> ()
                          }
                          frame #1 {
                            n811 = call "Save data file (stop) v3.vi"("panel id"=w1415) -> ("network file save error"=w1414:errorcluster)  [unwired: 9 in, 1 out]
                            n812 = local write "RESULT LAB03-2"(FALSE) -> ()
                            n813 = local write "data file error"(w1414) -> ()
                          }
                        }
                        n814 = Bundle(cluster=w1411, "STATUS"="STOP") -> (w1409:T4)  [unwired: 2 in]
                        n815 = local write "DISP LAB03-2"(w1409) -> ()
                      }
                    }
                  }
                  frame True {
                    n816 = local read "SIG LAB03-2"() -> (w1418:T2)
                    n817 = stacked-sequence {
                      seq-local: [w1429 _] -> [_ w1433]
                      tunnel: w1427 -> [_ w1443]
                      tunnel: w1426 -> [_ w1442]
                      tunnel: w1425 -> [_ w1441]
                      tunnel: w1424 -> [_ w1440]
                      tunnel: w1423 -> [_ w1439]
                      tunnel: [_ w1438] -> w1422
                      tunnel: w1421 -> [_ w1437]
                      tunnel: w1420 -> [_ w1436]
                      tunnel: w1419 -> [_ w1435]
                      tunnel: w1418 -> [w1428 w1434]
                      tunnel: w1417 -> [_ w1432]
                      frame #0 {
                        n818 = Unbundle(w1428) -> ("AMPS"=w1431:dbl)  [unwired: 4 out]
                        n819 = call "Check For Amps on v1.vi"("ID"="LAB03-2", "amps"=w1431) -> ("amps"=w1429:bool)  [unwired: 9 in]
                      }
                      frame #1 {
                        n820 = case shown="True" w1433 {
                          tunnel: w1443 -> [_ w1456]
                          tunnel: w1442 -> [_ w1455]
                          tunnel: w1441 -> [_ w1454]
                          tunnel: w1440 -> [_ w1453]
                          tunnel: w1439 -> [_ w1452]
                          tunnel: [errorcluster {"status"=FALSE, "code"=0, "source"=""} ("error out") w1451] -> w1438
                          tunnel: w1437 -> [_ w1450]
                          tunnel: w1436 -> [_ w1449]
                          tunnel: w1435 -> [_ w1448]
                          tunnel: w1434 -> [_ w1447]
                          tunnel: w1432 -> [_ w1446]
                          frame False {
                            w1444 = FALSE
                            n821 = local write "RUN LAB03-2"(w1444) -> ()
                            n822 = local write "run lab03-2"(w1444) -> ()
                          }
                          frame True {
                            n823 = stacked-sequence {
                              seq-local: [w1457 _ _ _ _] -> [_ w1481 _ _ _]
                              tunnel: w1456 -> [w1462 _ _ _ _]
                              tunnel: w1455 -> [w1459 _ _ _ _]
                              tunnel: w1454 -> [w1472 _ _ _ _]
                              tunnel: w1453 -> [w1465 _ _ _ _]
                              tunnel: w1452 -> [w1460 _ _ _ _]
                              tunnel: [_ w1476 _ _ _] -> w1451
                              tunnel: w1450 -> [_ _ _ w1502 _]
                              tunnel: w1449 -> [_ _ _ w1501 _]
                              tunnel: w1448 -> [_ _ _ w1500 _]
                              tunnel: w1447 -> [_ _ _ _ _]
                              tunnel: w1446 -> [_ _ _ _ w1516]
                              frame #0 {
                                w1458 = "\\"
                                n824 = local read "SET LAB03-2"() -> (w1467:T5)
                                n825 = case shown="\"T-RISE TEST\"" w1472 {
                                tunnel: ["L03-2-CHART TEST-" "L03-2-CYCLE TEST-" "L03-2-T-RISE TEST-"] -> w1468
                                frame "CHART TEST", Default {
                                }
                                frame "CYCLE TEST" {
                                }
                                frame "T-RISE TEST" {
                                }
                                }
                                n826 = Unbundle(w1467) -> ("DESCRIPTION"=w1466:string)  [unwired: 4 out]
                                n827 = Concatenate Strings(w1462, "\\", w1460, w1458, w1459, w1458) -> (w1469:string)
                                n828 = String To Path(string=w1469) -> (path=w1471:path)
                                n829 = Concatenate Strings(w1469, w1468, w1466, "-", w1465, ".tdms") -> (w1457:string)
                                n830 = Create Folder(path (use dialog)=w1471) -> (error out=w1470:errorcluster)  [unwired: 2 in, 2 out]
                                n831 = global write "Global 1.vi" "LAB03-2 FILE"(w1457) -> ()
                                n832 = call <vilib>:"Clear Errors.vi"("error in (no error)"=w1470) -> ()  [unwired: 5 in, 2 out]
                              }
                              frame #1 {
                                (unwired) FALSE
                                n833 = String To Path(string=w1481) -> (path=w1477:path)
                                n834 = TDMS Open(6:FALSE, 10:T21."create or replace" ("operation (0:open)"), 11:w1477) -> (0:w1476:errorcluster, 3:→"TDMS LAB03-2":refnum<k34>)  [unwired: 4 in]
                              }
                              frame #2 {
                                n835 = local read "SET LAB03-2"() -> (w1487:T5)
                                n836 = local read "TDMS LAB03-2"() -> (w1498:refnum<k34>)
                                n837 = Build Array("Testers Name", "Description", "Set Test Cycles", "T-Rise minutes", "T-Rise Deg C") -> (w1488:string[])
                                n838 = Unbundle(w1487) -> ("NAME"=w1486:string, "DESCRIPTION"=w1485:string, "CYCLES"=w1484:dbl, "T-RISE mins"=w1483:dbl, "T-RISE deg C"=w1482:dbl)
                                n839 = Number To Decimal String(number=w1484) -> (decimal integer string=w1497:string)  [unwired: 1 in]
                                n840 = Number To Decimal String(number=w1483) -> (decimal integer string=w1496:string)  [unwired: 1 in]
                                n841 = Number To Decimal String(number=w1482) -> (decimal integer string=w1495:string)  [unwired: 1 in]
                                n842 = Build Array(w1486, w1485, w1497, w1496, w1495) -> (w1494:string[])
                                n843 = TDMS Set Properties(5:w1494, 7:w1488, 11:w1498) -> ()  [unwired: 3 in, 4 out]
                              }
                              frame #3 {
                                n844 = local read "DISP LAB03-2"() -> (w1503:T4)
                                n845 = Concatenate Strings("LAB03-2  ", w1502) -> (w1504:string)
                                n846 = Two Button Dialog(message=w1504, 1:w1500, 2:w1501) -> (T button?=w1506:bool)
                                n847 = case shown="True" w1506 {
                                tunnel: w1503 -> [w1513 w1514]
                                tunnel: [w1513 w1514] -> w1510
                                tunnel: [w1512 w1515] -> w1509
                                tunnel: [w1511 w1515] -> w1508
                                frame False {
                                n848 = Unbundle(w1513) -> ("CYCLE"=w1512:dbl, "MINS"=w1511:dbl)  [unwired: 1 out]
                                }
                                frame True {
                                w1515 = 0.0
                                }
                                }
                                n849 = Bundle(cluster=w1510, "CYCLE"=w1509, "MINS"=w1508, "STATUS"="RUN") -> (w1499:T4)
                                n850 = local write "DISP LAB03-2"(w1499) -> ()
                              }
                              frame #4 {
                                n851 = local read "TEMP START LAB03-2"() -> (w1518:cluster{"TL":dbl, "TN":dbl})
